vi "ShowSwitchCurs.vi"(9 "Visible names?":bool=TRUE, 10 "All Lines":T2, 11 "Map":refnum<vi>) -> (3 "Map out":refnum<vi>, 4 "Switch Op":T1[](array[typedef]))   [LabVIEW 2014]
uses:
  Libraries/Map Data Folder/All-Lines.ctl
  Libraries/Map Data Folder/LineCluster.ctl
  Libraries/Map Data Folder/LineConnection.ctl
  Components/AutoMapBuilder/Conrtols/SwitchOp.ctl
  Libraries/Map Data Folder/Map Data.lvlib
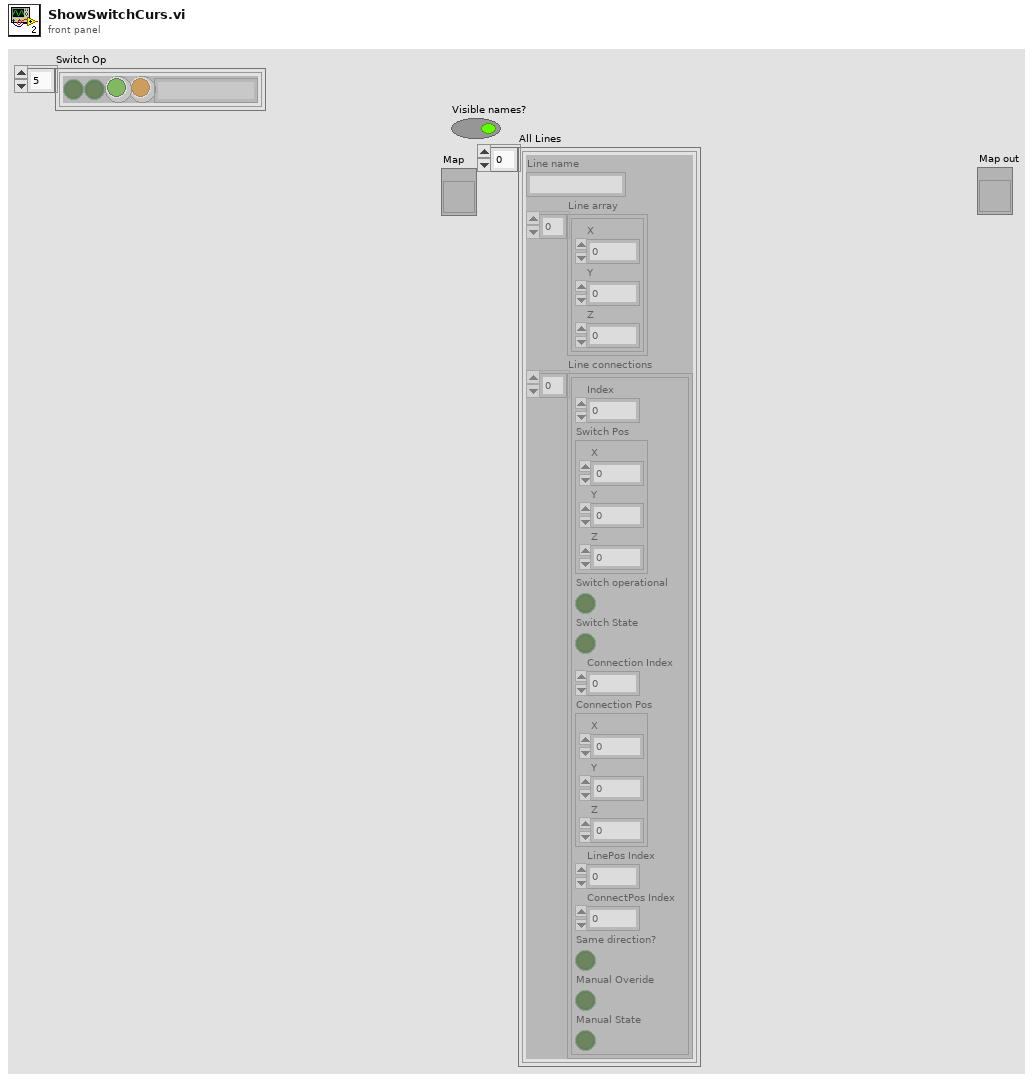
[diagram p1: front panel]
types:
  T1 = typedef "SwitchOp.ctl" = cluster{"Switch operational":bool, "Switch State":bool, "Manual Overide":bool, "Manual State":bool, "Switch\nPosition":cluster{"X":dbl, "Y":dbl, "Z":dbl}, "Index":i32, "Connection Index":i32, "Switch Index":i32, string}
  T2 = typedef "Map Data.lvlib/All-Lines.ctl" = T3[]
  T3 = typedef "Map Data.lvlib/LineCluster.ctl" = cluster{"Line name":string, "Line array":cluster{"X":dbl, "Y":dbl, "Z":dbl}[], "Line connections":T4[]}
  T4 = typedef "LineConnection.ctl" = cluster{"Index":i32, "Switch Pos":cluster{"X":dbl, "Y":dbl, "Z":dbl}, "Switch operational":bool, "Switch State":bool, "Connection Index":i32, "Connection Pos":cluster{"X":dbl, "Y":dbl, "Z":dbl}, "LinePos Index":i32, "ConnectPos Index":i32, "Same direction?":bool, "Manual Overide":bool, "Manual State":bool}
  T5 = typedef "LVCursorListTypeDef.ctl" = cluster{"Name":string, "Color":u32, "Style":u8, "Point Style":u8, "Name Visible":bool, "Allow Drag":bool, "Cursor Mode":u32, "Plot":i32, "Index":i32, "Position":cluster{"X":dbl, "Y":dbl}, "X Scale":u32, "Y Scale":u32, "Watch Plots":i32[], "Watch All Plots":bool, "Plot Area":i32, "Label Offset":cluster{"X":dbl, "Y":dbl}}[]
  T6 = cluster{"Name":string, "Color":u32, "Style":u8, "Point Style":u8, "Name Visible":bool, "Allow Drag":bool, "Cursor Mode":u32, "Plot":i32, "Index":i32, "Position":cluster{"X":dbl, "Y":dbl}, "X Scale":u32, "Y Scale":u32, "Watch Plots":i32[], "Watch All Plots":bool, "Plot Area":i32, "Label Offset":cluster{"X":dbl, "Y":dbl}}
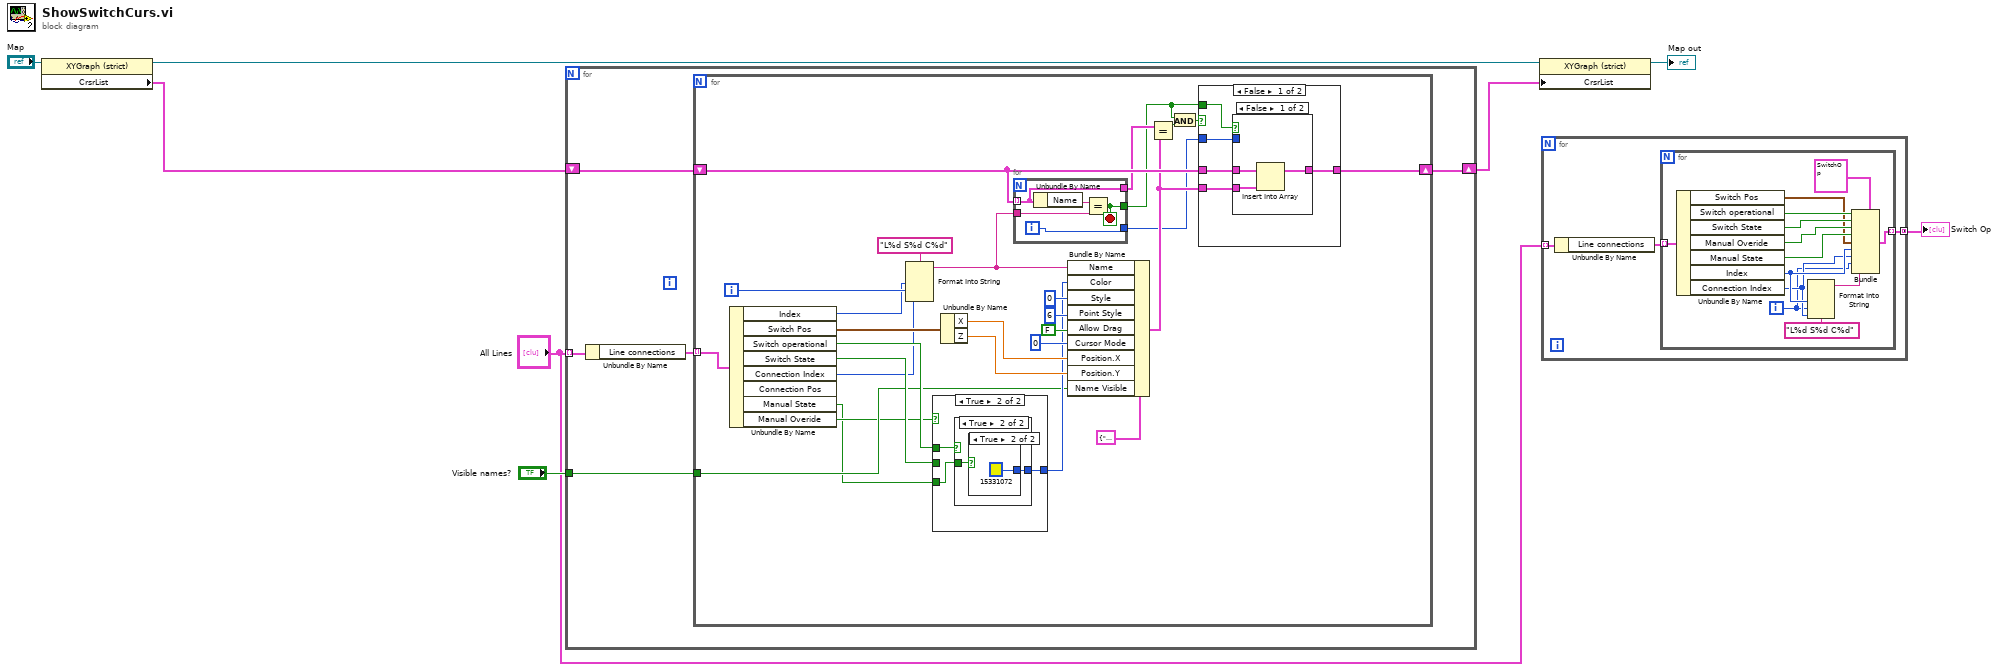
[diagram p0: block diagram]
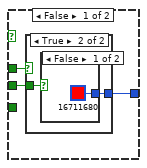
[diagram p2: hidden frame]
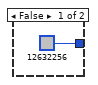
[diagram p3: hidden frame]
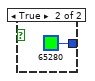
[diagram p4: hidden frame]
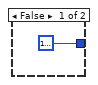
[diagram p5: hidden frame]
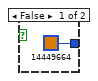
[diagram p6: hidden frame]
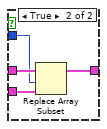
[diagram p7: hidden frame]
diagram:
  n1 = property on="Property Node" class="XYGraph (strict)"(reference="Map") -> (reference out=w6:refnum<vi>, "CrsrList"=w5:T5)  [unwired: 1 in, 1 out]
  n2 = for {
    tunnel: "All Lines" -> [w13] mode=indexing
    shift-right: [w11] -> w3
    shift-left: w5 -> [w10]
    tunnel: "Visible names?" -> [w9]
    n3 = Unbundle By Name(w13) -> ("Line connections"=w12:T4[])
    n4 = for {
      tunnel: w12 -> [w41] mode=indexing
      shift-right: [w25] -> w11
      shift-left: w10 -> [w24]
      tunnel: w9 -> [w19]
      i -> [w17]
      n5 = Unbundle By Name(w41) -> ("Index"=w14:i32, "Switch Pos"=w40:cluster{"X":dbl, "Y":dbl, "Z":dbl}, "Switch operational"=w31:bool, "Switch State"=w30:bool, "Connection Index"=w18:i32, "Manual State"=w15:bool, "Manual Overide"=w16:bool)  [unwired: 1 out]
      n6 = Format Into String(format string="L%d S%d C%d", w14, w17, w18) -> (resulting string=w28:string)  [unwired: 2 in, 1 out]
      n7 = case shown="True" w16 {
        tunnel: w31 -> [w44 w51]
        tunnel: w30 -> [w43 _]
        tunnel: [w42 w52] -> w29
        tunnel: w15 -> [_ w50]
        frame False {
          n8 = case shown="True" w44 {
            tunnel: w43 -> [_ w47]
            tunnel: [u32 12632256 w46] -> w42
            frame False {
            }
            frame True {
              n9 = case shown="False" w47 {
                tunnel: [u32 16711680 u32 65280] -> w46
                frame False {
                }
                frame True {
                }
              }
            }
          }
        }
        frame True {
          n10 = case shown="True" w51 {
            tunnel: w50 -> [_ w55]
            tunnel: [u32 16777222 w54] -> w52
            frame False {
            }
            frame True {
              n11 = case shown="True" w55 {
                tunnel: [u32 14449664 u32 15331072] -> w54
                frame False {
                }
                frame True {
                }
              }
            }
          }
        }
      }
      n12 = Unbundle By Name(w40) -> ("X"=w39:dbl, "Z"=w38:dbl)
      n13 = for {
        tunnel: w24 -> [w71] mode=indexing
        tunnel: w28 -> [w75]
        tunnel: [w73] -> w20
        tunnel: [w72] -> w21
        tunnel: [w71] -> w22
        i -> [w72]
        stop <- w73 stop-if-true
        n14 = Unbundle By Name(w71) -> ("Name"=w74:string)
        n15 = Equal?(x=w74, y=w75) -> (x = y?=w73:bool)
      }
      n16 = Bundle By Name(cluster=T6 {"Name"="Cursor 1", "Color"=16777222, "Style"=0, "Point Style"=6, "Name Visible"=TRUE, "Allow Drag"=TRUE, "Cursor Mode"=0, "Plot"=0, "Index"=0, "Position"={"X"=-7.216103869606, "Y"=403.5}, "X Scale"=0, "Y Scale"=0, "Watch Plots"=[], "Watch All Plots"=FALSE, "Plot Area"=0, "Label Offset"={"X"=-0.0029596755445018275, "Y"=-0.588709677419331}}, "Name"=w28, "Color"=w29, "Style"=u8 0, "Point Style"=u8 6, "Allow Drag"=FALSE, "Cursor Mode"=u32 0, "Position.X"=w39, "Position.Y"=w38, "Name Visible"=w19) -> (w23:T6)
      n17 = Equal?(x=w22, y=w23) -> (x = y?=w26:bool)
      n18 = And(x=w20, y=w26) -> (x .and. y?=w27:bool)
      n19 = case shown="False" w27 {
        tunnel: [w62 w70] -> w25
        tunnel: w23 -> [w60 _]
        tunnel: w24 -> [w61 w70]
        tunnel: w21 -> [w59 _]
        tunnel: w20 -> [w58 _]
        frame False {
          n20 = case shown="False" w58 {
            tunnel: [w64 w69] -> w62
            tunnel: w61 -> [w65 w68]
            tunnel: w60 -> [w63 w67]
            tunnel: w59 -> [_ w66]
            frame False {
              n21 = Insert Into Array(array=w65, new element=w63) -> (w64:T5)  [unwired: 1 in]
            }
            frame True {
              n22 = Replace Array Subset(array=w68, new element=w67, index=w66) -> (w69:T5)
            }
          }
        }
        frame True {
        }
      }
    }
  }
  n23 = property on="Property Node" class="XYGraph (strict)"(reference=w6, "CrsrList"=w3) -> (reference out=→"Map out":refnum<vi>)  [unwired: 1 in, 1 out]
  n24 = for {
    tunnel: "All Lines" -> [w78] mode=indexing
    tunnel: [w76] -> w1 mode=concatenating
    n25 = Unbundle By Name(w78) -> ("Line connections"=w77:T4[])
    n26 = for {
      tunnel: w77 -> [w91] mode=indexing
      tunnel: [w89] -> w76 mode=indexing
      i -> [w79]
      n27 = Unbundle By Name(w91) -> ("Switch Pos"=w83:cluster{"X":dbl, "Y":dbl, "Z":dbl}, "Switch operational"=w87:bool, "Switch State"=w86:bool, "Manual Overide"=w85:bool, "Manual State"=w84:bool, "Index"=w82:i32, "Connection Index"=w81:i32)
      n28 = Format Into String(format string="L%d S%d C%d", w82, w79, w81) -> (resulting string=w80:string)  [unwired: 2 in, 1 out]
      n29 = Bundle(cluster=T1 {"Switch operational"=FALSE, "Switch State"=FALSE, "Manual Overide"=FALSE, "Manual State"=FALSE, "Switch\nPosition"={"X"=1401.4972181059047, "Y"=55.368, "Z"=5623.149736695605}, "Index"=0, "Connection Index"=3, "Switch Index"=0, "L0 S0 C3"}, "Switch operational"=w87, "Switch State"=w86, "Manual Overide"=w85, "Manual State"=w84, "Switch\nPosition"=w83, "Index"=w82, "Connection Index"=w81, "Switch Index"=w79, w80) -> (w89:T1)
    }
  }
  "Switch Op" <- w1
